vi "UI.vi"() -> ()   [LabVIEW 2018]
uses:
  data/MyControlAll.dll
panel:
  in  "多语言测试":refnum<k24>(container)
  in  "双击选中":refnum<k24>(container)
  in  "单击选中":refnum<k24>(container)
  in  "TreePanel":refnum<k24>(container)
  in  "按钮颜色":u32(colorbox)
  in  "渐变终点":u32(colorbox)
  in  "渐变起点":u32(colorbox)
  in  "ButtonPanel 10":refnum<k24>(container)
  in  "ButtonPanel 9":refnum<k24>(container)
  in  "开关":refnum<k24>(container)
  in  "文本":refnum<k24>(container)
  in  "滑动杆":refnum<k24>(container)
  in  "进度条":refnum<k24>(container)
  in  "ButtonPanel 4":refnum<k24>(container)
  in  "ButtonPanel 3":refnum<k24>(container)
  in  "ButtonPanel 2":refnum<k24>(container)
  in  "ButtonPanel":refnum<k24>(container)
  in  "ChartPanel":refnum<k24>(container)
  in  "DataGridPanel":refnum<k24>(container)
  in  "ButtonPanel 12":refnum<k24>(container)
  in  "ButtonPanel 11":refnum<k24>(container)
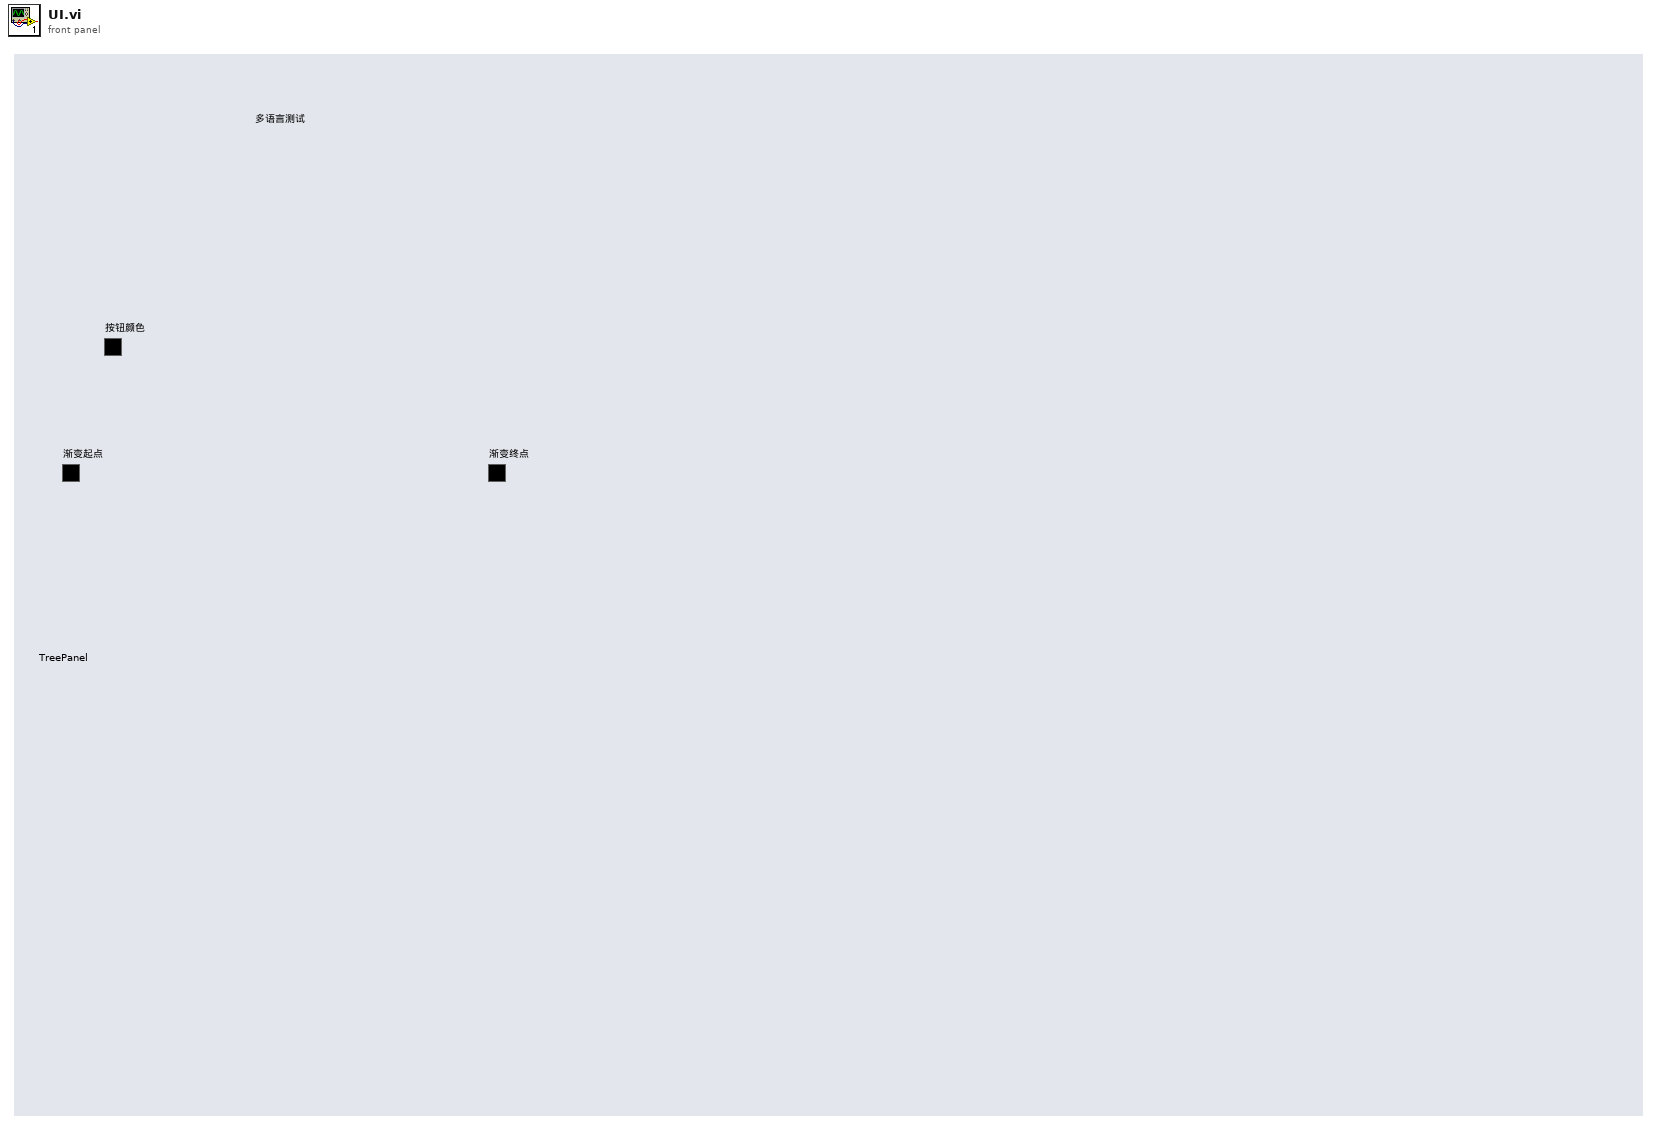
[diagram p1: front panel]
types:
  T1 = cluster{"selectedIndex":i32, "selectedItem":string, "selectedItemUTF8":u8[]}
  T2 = cluster{"nodeId":string, "nodeText":string, "nodeTextUTF8":u8[]}
  T3 = cluster{"id":string, "parentId":string, "text":string, "isChecked":bool, "showCheckBox":bool, "hasDummyChild":bool, "iconPath":string}[]
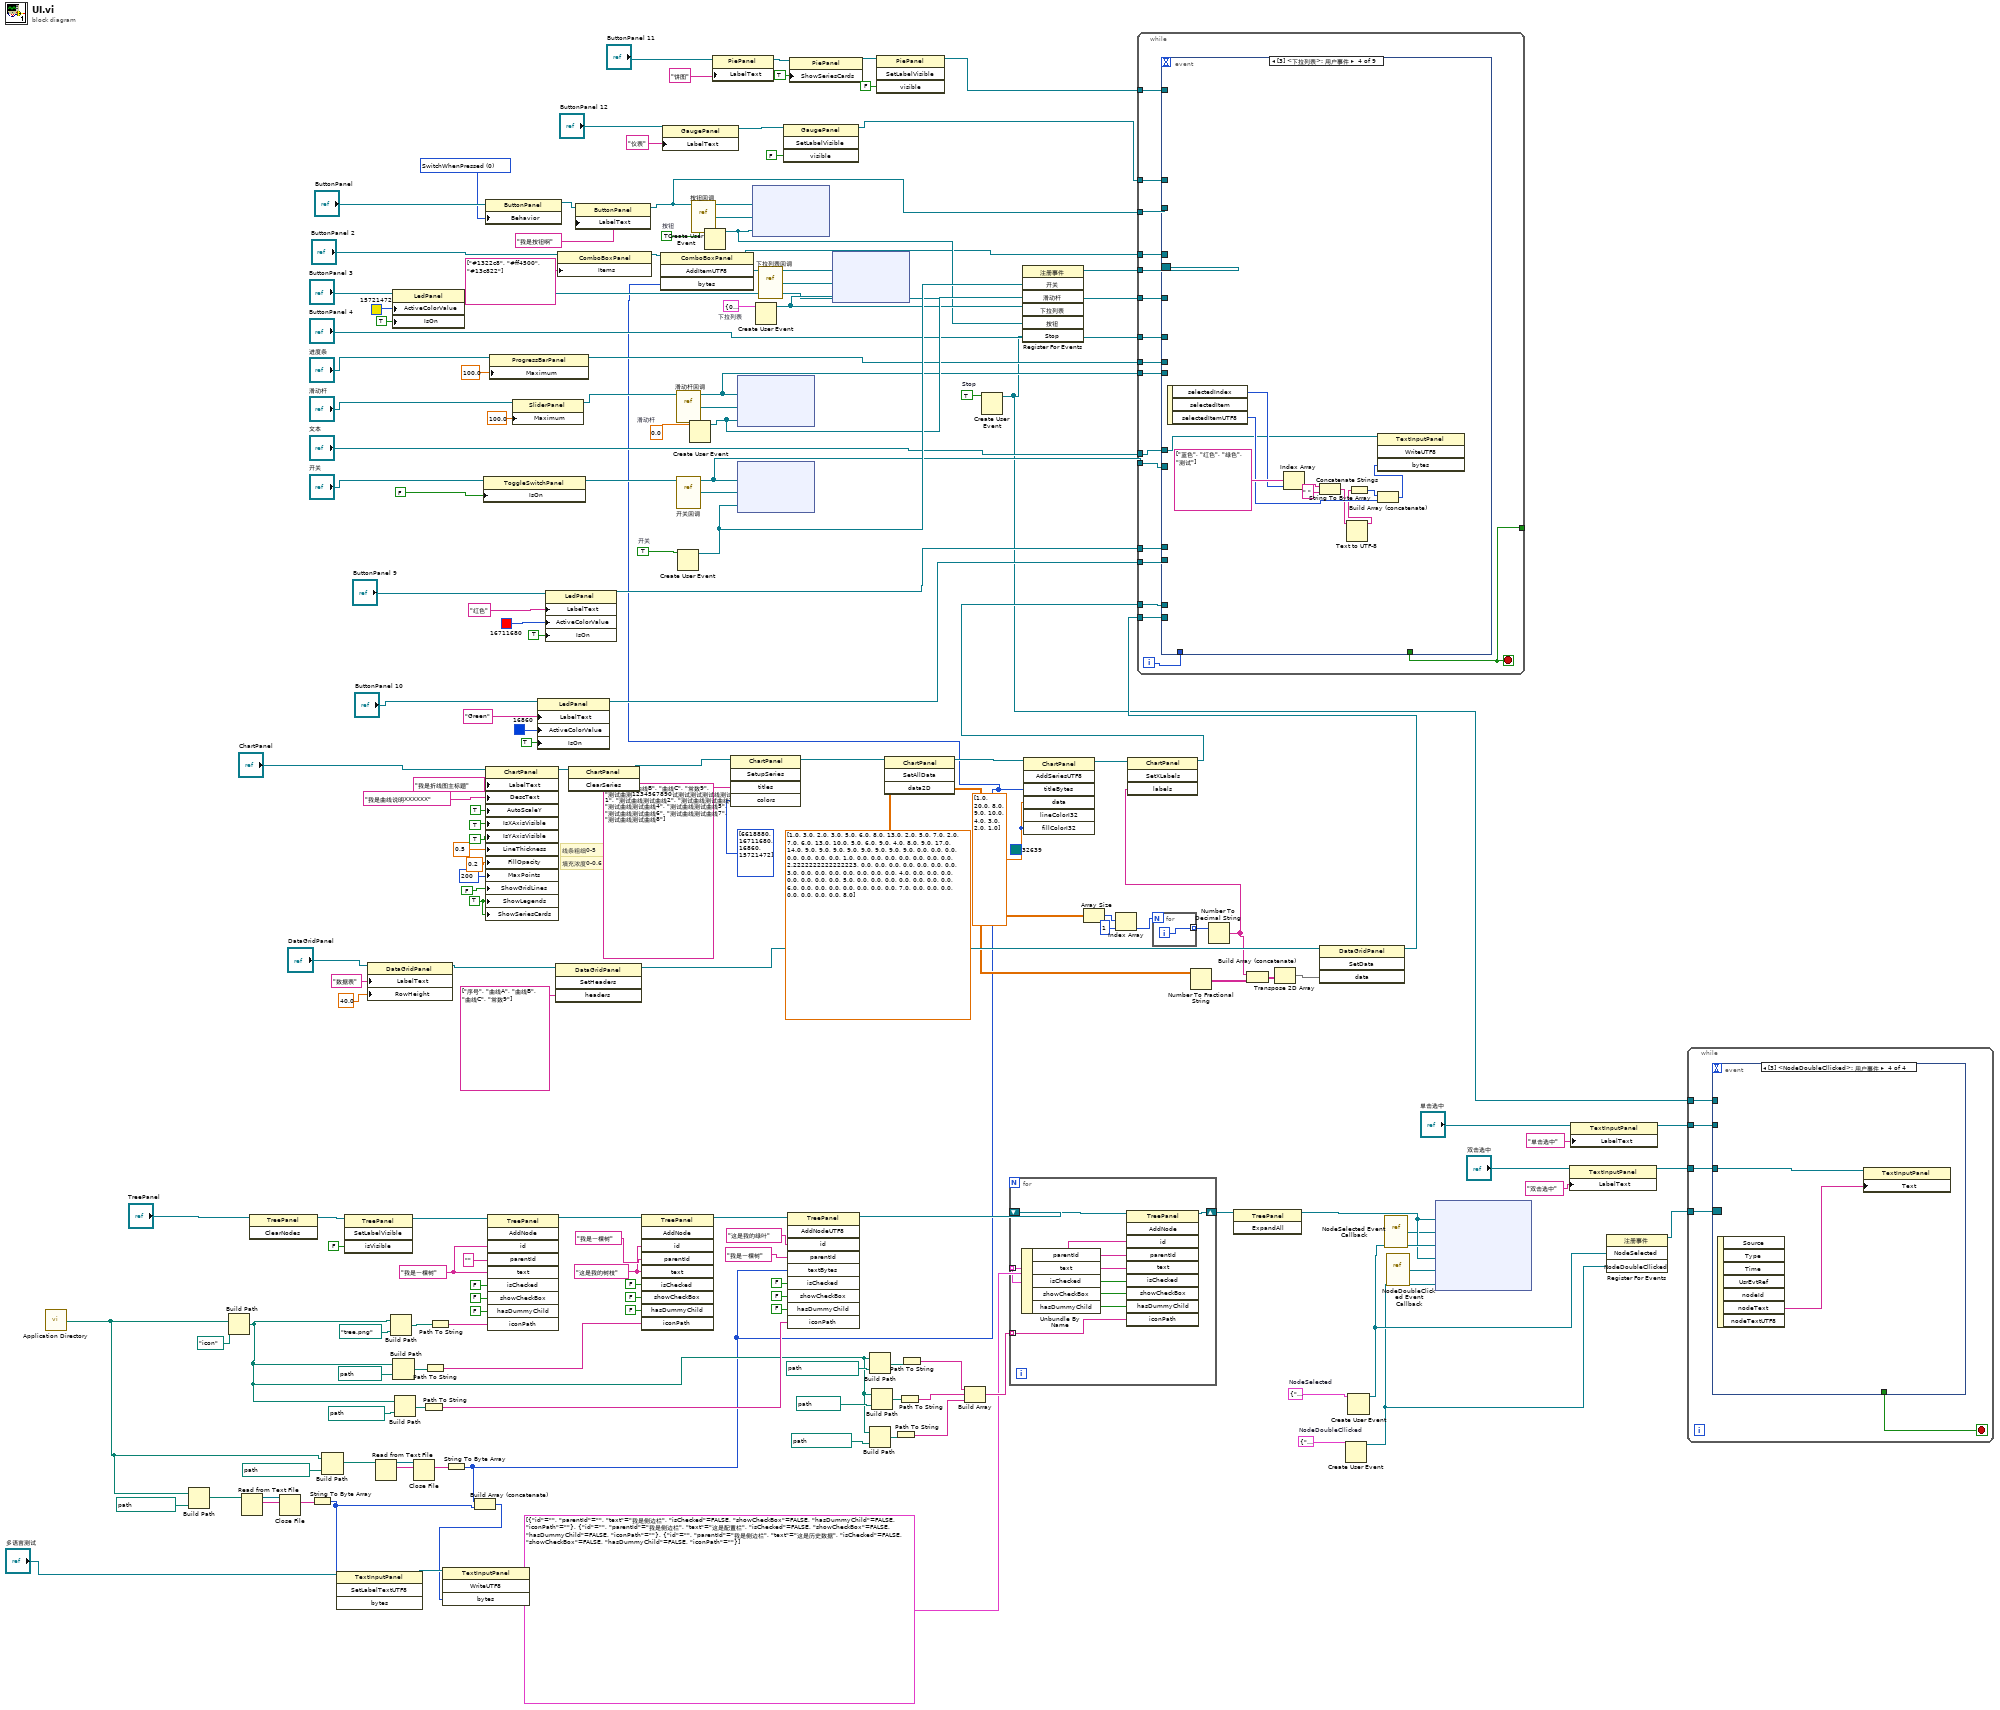
[diagram p0: block diagram]
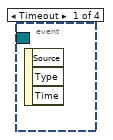
[diagram p2: hidden frame]
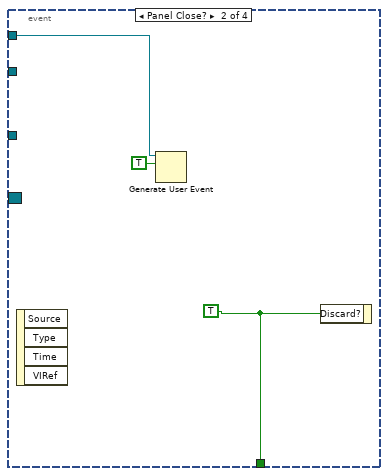
[diagram p3: hidden frame]
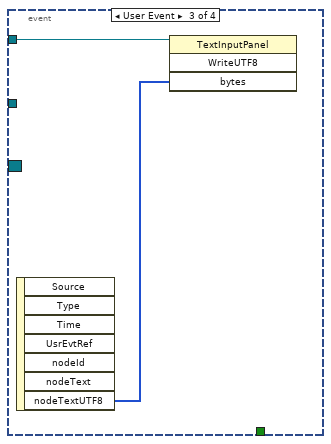
[diagram p4: hidden frame]
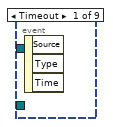
[diagram p5: hidden frame]
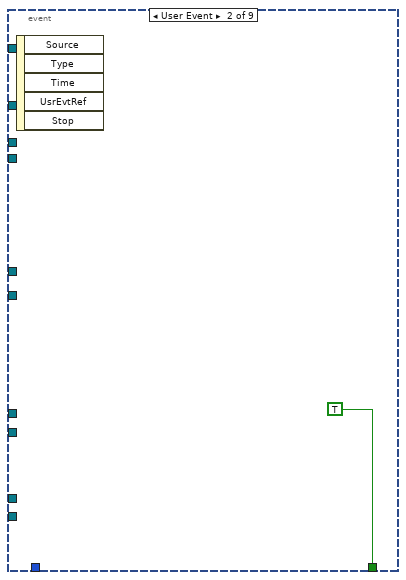
[diagram p6: hidden frame]
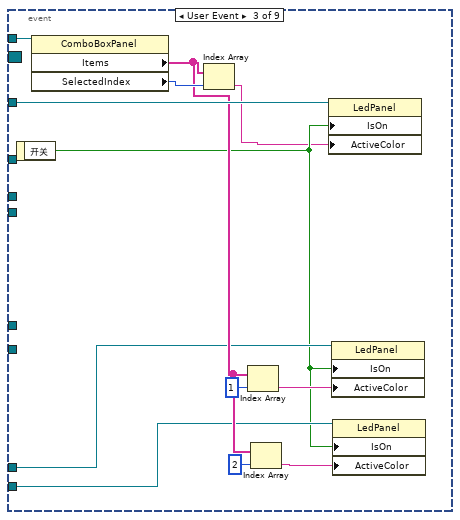
[diagram p7: hidden frame]
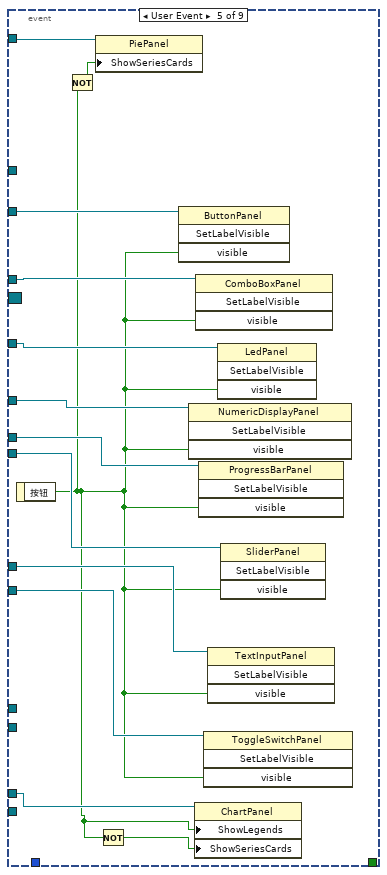
[diagram p8: hidden frame]
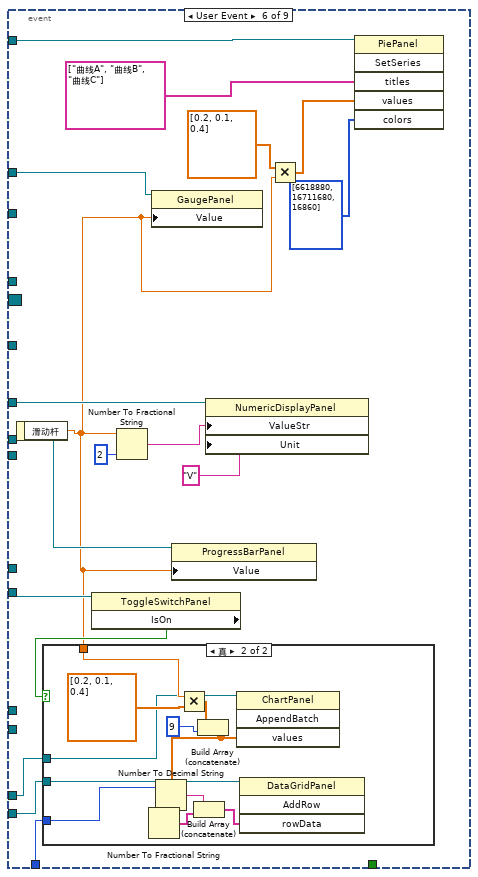
[diagram p9: hidden frame]
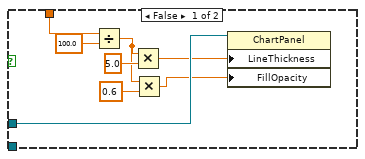
[diagram p10: hidden frame]
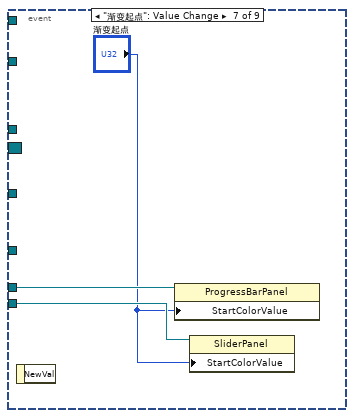
[diagram p11: hidden frame]
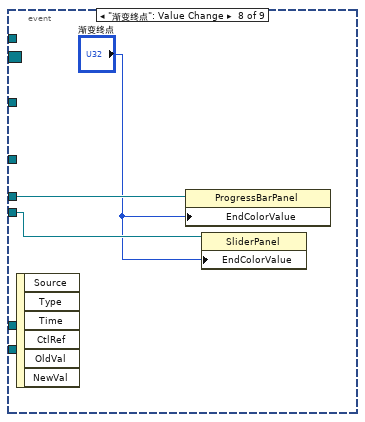
[diagram p12: hidden frame]
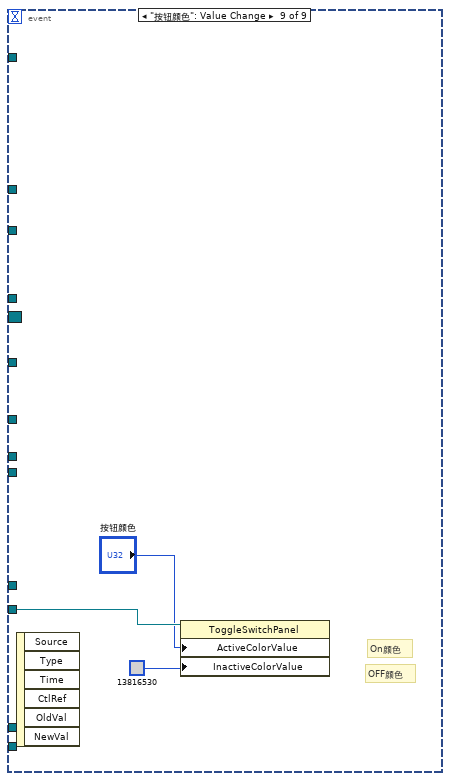
[diagram p13: hidden frame]
diagram:
  w3 = u32 32639
  w8 = T1 {"selectedIndex"=0, "selectedItem"="", "selectedItemUTF8"=[]}  # 下拉列表
  w11 = T2 {"nodeId"="", "nodeText"="", "nodeTextUTF8"=[]}  # NodeDoubleCllicked
  w12 = T2 {"nodeId"="", "nodeText"="", "nodeTextUTF8"=[]}  # NodeSelected
  w37 = TRUE  # Stop
  w63 = "这是我的树枝" ("text")
  w65 = "我是一棵树" ("text")
  w102 = TRUE ("ShowLegends")
  w141 = 0 items=["SwitchWhenPressed", "SwitchWhenReleased", "SwitchUntilReleased", "LatchWhenPressed", "LatchWhenReleased"] ("Behavior")
  w146 = TRUE  # 按钮
  w161 = 0.0  # 滑动杆
  w170 = TRUE  # 开关
  # "填充浓度0-0.6"
  # "线条粗细0-5"
  n1 = call <vilib>:"Application Directory.vi"() -> ("Application Directory"=w16:path)
  n2 = Build Path(base path=w16, name or relative path=path "data/韩文.txt" ("路径")) -> (appended path=w18:path)
  n3 = Build Path(base path=w16, name or relative path=path "icon" ("路径")) -> (appended path=w25:path)
  n4 = Read from Text File(file (use dialog)=w18) -> (refnum out=w20:refnum<file>, text=w19:string)  [unwired: 3 in, 2 out]
  n5 = invoke on="调用节点" class="TreePanel" method="ClearNodes"(reference="TreePanel") -> (reference out=w61:refnum<k24>)  [unwired: 2 in, 2 out]
  n6 = Close File(refnum=w20) -> ()  [unwired: 1 in, 2 out]
  n7 = String To Byte Array(string=w19) -> (unsigned byte array=w14:u8[])
  n8 = Build Path(base path=w16, name or relative path=path "data/越南文.txt" ("路径")) -> (appended path=w24:path)
  n9 = invoke on="调用节点" class="TextInputPanel" method="SetLabelTextUTF8"(reference="多语言测试", "bytes"=w14) -> (reference out=w15:refnum<k24>)  [unwired: 2 in, 3 out]
  n10 = invoke on="调用节点" class="TreePanel" method="SetLabelVisible"(reference=w61, "isVisible"=FALSE) -> (reference out=w59:refnum<k24>)  [unwired: 2 in, 3 out]
  n11 = property on="属性节点" class="DataGridPanel"(reference="DataGridPanel", "LabelText"="数据表", "RowHeight"=40.0) -> (reference out=w130:refnum<k24>)  [unwired: 1 in, 1 out]
  n12 = Read from Text File(file (use dialog)=w24) -> (refnum out=w22:refnum<file>, text=w23:string)  [unwired: 3 in, 2 out]
  n13 = Build Path(base path=w25, name or relative path=path "tree.png" ("路径")) -> (appended path=w48:path)
  n14 = property on="属性节点" class="LedPanel"(reference="ButtonPanel 3", "ActiveColorValue"=u32 15721472, "IsOn"=TRUE) -> (reference out=w97:refnum<k24>)  [unwired: 1 in, 1 out]
  n15 = Build Path(base path=w25, name or relative path=path "树枝.png" ("路径")) -> (appended path=w46:path)
  n16 = Build Path(base path=w25, name or relative path=path "绿叶 (1).png" ("路径")) -> (appended path=w44:path)
  n17 = Close File(refnum=w22) -> ()  [unwired: 1 in, 2 out]
  n18 = Path To String(path=w44) -> (string=w68:string)
  n19 = Path To String(path=w46) -> (string=w67:string)
  n20 = Path To String(path=w48) -> (string=w73:string)
  n21 = String To Byte Array(string=w23) -> (unsigned byte array=w1:u8[])
  n22 = Build Array (concatenate)(w1, w14) -> (w13:u8[])
  n23 = invoke on="调用节点" class="TextInputPanel" method="WriteUTF8"(reference=w15, "bytes"=w13) -> ()  [unwired: 2 in, 4 out]
  n24 = property on="属性节点" class="ToggleSwitchPanel"(reference="开关", "IsOn"=FALSE) -> (reference out=w140:refnum<k24>)  [unwired: 1 in, 1 out]
  n25 = property on="属性节点" class="ButtonPanel"(reference="ButtonPanel", "Behavior"=w141) -> (reference out=w138:refnum<k24>)  [unwired: 1 in, 1 out]
  n26 = property on="属性节点" class="ChartPanel"(reference="ChartPanel", "LabelText"="我是折线图主标题", "DescText"="我是曲线说明XXXXXX", "AutoScaleY"=TRUE, "IsXAxisVisible"=TRUE ("AutoScaleY"), "IsYAxisVisible"=TRUE ("AutoScaleY"), "LineThickness"=0.5, "FillOpacity"=0.2, "MaxPoints"=200, "ShowGridLines"=FALSE, "ShowLegends"=w102, "ShowSeriesCards"=w102) -> (reference out=w125:refnum<k24>)  [unwired: 1 in, 1 out]
  n27 = invoke on="调用节点" class="TreePanel" method="AddNode"(reference=w59, "id"=w65, "parentId"="", "text"=w65, "isChecked"=FALSE, "showCheckBox"=FALSE, "hasDummyChild"=FALSE, "iconPath"=w73) -> (reference out=w77:refnum<k24>)  [unwired: 2 in, 9 out]
  n28 = property on="属性节点" class="ProgressBarPanel"(reference="进度条", "Maximum"=100.0) -> (reference out=w155:refnum<k24>)  [unwired: 1 in, 1 out]
  n29 = property on="属性节点" class="SliderPanel"(reference="滑动杆", "Maximum"=100.0) -> (reference out=w139:refnum<k24>)  [unwired: 1 in, 1 out]
  n30 = property on="属性节点" class="LedPanel"(reference="ButtonPanel 10", "LabelText"="Green", "ActiveColorValue"=u32 16860, "IsOn"=TRUE) -> (reference out=w147:refnum<k24>)  [unwired: 1 in, 1 out]
  n31 = property on="属性节点" class="LedPanel"(reference="ButtonPanel 9", "LabelText"="红色", "ActiveColorValue"=u32 16711680, "IsOn"=TRUE) -> (reference out=w149:refnum<k24>)  [unwired: 1 in, 1 out]
  n32 = invoke on="调用节点" class="DataGridPanel" method="SetHeaders"(reference=w130, "headers"=string[] ["序号", "曲线A", "曲线B", "曲线C", "常数9"]) -> (reference out=w133:refnum<k24>)  [unwired: 2 in, 3 out]
  n33 = property class="ComboBoxPanel"(reference="ButtonPanel 2", "Items"=string[] ["#1322c8", "#ff4500", "#13c822"]) -> (reference out=w154:refnum<k24>)  [unwired: 1 in, 1 out]
  n34 = invoke on="调用节点" class="ChartPanel" method="ClearSeries"(reference=w125) -> (reference out=w111:refnum<k24>)  [unwired: 2 in, 2 out]
  n35 = property on="属性节点" class="ButtonPanel"(reference=w138, "LabelText"="我是按钮啊") -> (reference out=w137:refnum<k24>)  [unwired: 1 in, 1 out]
  n36 = invoke on="调用节点" class="TreePanel" method="AddNode"(reference=w77, "id"=w63, "parentId"="我是一棵树" ("text"), "text"=w63, "isChecked"=FALSE, "showCheckBox"=FALSE, "hasDummyChild"=FALSE, "iconPath"=w67) -> (reference out=w69:refnum<k24>)  [unwired: 2 in, 9 out]
  n37 = invoke on="调用节点" class="ComboBoxPanel" method="AddItemUTF8"(reference=w154, "bytes"=w1) -> (reference out=w2:refnum<k24>)  [unwired: 2 in, 3 out]
  n38 = property on="属性节点" class="GaugePanel"(reference="ButtonPanel 12", "LabelText"="仪表") -> (reference out=w90:refnum<k24>)  [unwired: 1 in, 1 out]
  n39 = vi-ref "滑动杆回调.vi"() -> ("vi reference"=w160:refnum<vi>)
  n40 = vi-ref "开关回调.vi"() -> ("vi reference"=w167:refnum<vi>)
  n41 = Create User Event(user event datatype=w170) -> (user event=w168:refnum<user-event>)  [unwired: 1 in, 1 out]
  n42 = Create User Event(user event datatype=w161) -> (user event=w159:refnum<user-event>)  [unwired: 1 in, 1 out]
  n43 = vi-ref "按钮回调.vi"() -> ("vi reference"=w144:refnum<vi>)
  n44 = Create User Event(user event datatype=w146) -> (user event=w143:refnum<user-event>)  [unwired: 1 in, 1 out]
  n45 = property on="属性节点" class="PiePanel"(reference="ButtonPanel 11", "LabelText"="饼图") -> (reference out=w85:refnum<k24>)  [unwired: 1 in, 1 out]
  n46 = invoke on="调用节点" class="ChartPanel" method="SetupSeries"(reference=w111, "titles"=string[] ["曲线A", "曲线B", "曲线C", "常数9", "测试曲测1234567890试测试测试测试线测试曲线1", "测试曲线测试曲线2", "测试曲线测试曲线3", "测试曲线测试曲线4", "测试曲线测试曲线5", "测试曲线测试曲线6", "测试曲线测试曲线7", "测试曲线测试曲线8"], "colors"=u32[] [6618880, 16711680, 16860, 15721472]) -> (reference out=w110:refnum<k24>)  [unwired: 2 in, 4 out]
  n47 = node(w139, w160, w159) -> ()  [unwired: 2 in, 2 out]
  n48 = node(w140, w167, w168) -> ()  [unwired: 2 in, 2 out]
  n49 = node(w137, w144, w143) -> ()  [unwired: 2 in, 2 out]
  n50 = Create User Event(user event datatype=w8) -> (user event=w153:refnum<user-event>)  [unwired: 1 in, 1 out]
  n51 = vi-ref "下拉列表回调.vi"() -> ("vi reference"=w7:refnum<vi>)
  n52 = invoke on="调用节点" class="GaugePanel" method="SetLabelVisible"(reference=w90, "visible"=FALSE) -> (reference out=w89:refnum<k24>)  [unwired: 2 in, 3 out]
  n53 = invoke on="调用节点" class="TreePanel" method="AddNodeUTF8"(reference=w69, "id"="这是我的绿叶" ("text"), "parentId"="我是一棵树" ("text"), "textBytes"=w1, "isChecked"=FALSE, "showCheckBox"=FALSE, "hasDummyChild"=FALSE, "iconPath"=w68) -> (reference out=w66:refnum<k24>)  [unwired: 2 in, 9 out]
  n54 = property on="属性节点" class="PiePanel"(reference=w85, "ShowSeriesCards"=TRUE) -> (reference out=w84:refnum<k24>)  [unwired: 1 in, 1 out]
  n55 = node(w2, w7, w153) -> ()  [unwired: 2 in, 2 out]
  n56 = Build Path(base path=w25, name or relative path=path "历史数据.png" ("路径")) -> (appended path=w38:path)
  n57 = Build Path(base path=w25, name or relative path=path "侧边栏_探索.png" ("路径")) -> (appended path=w42:path)
  n58 = Build Path(base path=w25, name or relative path=path "配置.png" ("路径")) -> (appended path=w40:path)
  n59 = invoke on="调用节点" class="PiePanel" method="SetLabelVisible"(reference=w84, "visible"=FALSE) -> (reference out=w87:refnum<k24>)  [unwired: 2 in, 3 out]
  n60 = invoke on="调用节点" class="ChartPanel" method="SetAllData"(reference=w110, "data2D"=dbl[][] [[1.0, 3.0, 2.0, 3.0, 5.0, 6.0, 8.0, 13.0], [2.0, 5.0, 7.0, 2.0, 7.0, 6.0, 13.0, 10.0], [5.0, 6.0, 9.0, 4.0, 8.0, 9.0, 17.0, 14.0], [9.0, 9.0, 9.0, 9.0, 9.0, 9.0, 9.0, 9.0], [0.0, 0.0, 0.0, 0.0, 0.0, 0.0, 0.0, 1.0], [0.0, 0.0, 0.0, 0.0, 0.0, 0.0, 0.0, 2.2222222222222223], [0.0, 0.0, 0.0, 0.0, 0.0, 0.0, 0.0, 3.0], [0.0, 0.0, 0.0, 0.0, 0.0, 0.0, 0.0, 4.0], [0.0, 0.0, 0.0, 0.0, 0.0, 0.0, 0.0, 5.0], [0.0, 0.0, 0.0, 0.0, 0.0, 0.0, 0.0, 6.0], [0.0, 0.0, 0.0, 0.0, 0.0, 0.0, 0.0, 7.0], [0.0, 0.0, 0.0, 0.0, 0.0, 0.0, 0.0, 8.0]]) -> (reference out=w6:refnum<k24>, "data2D"=w117:dbl[][])  [unwired: 2 in, 2 out]
  n61 = Path To String(path=w38) -> (string=w33:string)
  n62 = Path To String(path=w40) -> (string=w34:string)
  n63 = Path To String(path=w42) -> (string=w35:string)
  n64 = Build Array(w35, w34, w33) -> (w32:string[])
  n65 = Create User Event(user event datatype=w37) -> (user event=w36:refnum<user-event>)  [unwired: 1 in, 1 out]
  n66 = for {
    shift-right: [w180] -> w30
    shift-left: w66 -> [w181]
    tunnel: w32 -> [w179] mode=indexing
    tunnel: T3 [{"id"="", "parentId"="", "text"="我是侧边栏", "isChecked"=FALSE, "showCheckBox"=FALSE, "hasDummyChild"=FALSE, "iconPath"=""}, {"id"="", "parentId"="我是侧边栏", "text"="这是配置栏", "isChecked"=FALSE, "showCheckBox"=FALSE, "hasDummyChild"=FALSE, "iconPath"=""}, {"id"="", "parentId"="我是侧边栏", "text"="这是历史数据", "isChecked"=FALSE, "showCheckBox"=FALSE, "hasDummyChild"=FALSE, "iconPath"=""}] -> [w178] mode=indexing
    n67 = Unbundle By Name(w178) -> ("parentId"=w176:string, "text"=w177:string, "isChecked"=w175:bool, "showCheckBox"=w174:bool, "hasDummyChild"=w173:bool)
    n68 = invoke on="调用节点" class="TreePanel" method="AddNode"(reference=w181, "id"=w177, "parentId"=w176, "text"=w177, "isChecked"=w175, "showCheckBox"=w174, "hasDummyChild"=w173, "iconPath"=w179) -> (reference out=w180:refnum<k24>)  [unwired: 2 in, 9 out]
  }
  n69 = register-events(w168, w159, w153, w143, w36) -> (reference out=w169:refnum<event-registration>)  [unwired: 2 in, 1 out]
  n70 = invoke on="调用节点" class="ChartPanel" method="AddSeriesUTF8"(reference=w6, "titleBytes"=w1, "data"=dbl[] [1.0, 20.0, 8.0, 9.0, 10.0, 4.0, 3.0, 2.0, 1.0], "lineColorI32"=w3, "fillColorI32"=w3) -> (reference out=w5:refnum<k24>)  [unwired: 2 in, 6 out]
  n71 = Array Size(array=w117) -> (size(s)=w116:i32[])
  n72 = Index Array(array=w116, index=1 ("索引")) -> (element=w114:i32)
  n73 = for {
    N: w114 -> [_]
    tunnel: [w182] -> w113 mode=indexing
    i -> [w182]
  }
  n74 = Number To Fractional String(number=w117) -> (F-format string=w118:string[][])  [unwired: 3 in]
  n75 = Number To Decimal String(number=w113) -> (decimal integer string=w109:string[])  [unwired: 1 in]
  n76 = invoke on="调用节点" class="ChartPanel" method="SetXLabels"(reference=w5, "labels"=w109) -> (reference out=w108:refnum<k24>)  [unwired: 2 in, 3 out]
  n77 = invoke on="调用节点" class="TreePanel" method="ExpandAll"(reference=w30) -> (reference out=w29:refnum<k24>)  [unwired: 2 in, 2 out]
  n78 = Build Array (concatenate)(w109, w118) -> (w112:string[][])
  n79 = Transpose 2D Array(2D array=w112) -> (transposed array=w132:string[][])
  n80 = invoke on="调用节点" class="DataGridPanel" method="SetData"(reference=w133, "data"=w132) -> (reference out=w106:refnum<k24>)  [unwired: 2 in, 3 out]
  n81 = while {
    tunnel: w169 -> [w199]
    tunnel: w97 -> [w198]
    tunnel: w2 -> [w197]
    tunnel: "文本" -> [w196]
    tunnel: "ButtonPanel 4" -> [w195]
    tunnel: w155 -> [w194]
    tunnel: w149 -> [w193]
    tunnel: w147 -> [w192]
    tunnel: w137 -> [w191]
    tunnel: w140 -> [w190]
    tunnel: w139 -> [w189]
    tunnel: w108 -> [w188]
    tunnel: w106 -> [w187]
    tunnel: w89 -> [w185]
    tunnel: w87 -> [w184]
    tunnel: [w183] -> _
    i -> [w186]
    stop <- w183 stop-if-true
    n82 = event shown="[3] <下拉列表>: 用户事件" {
      selector: w199 -> [_ _ _ _ _ _ _ _ _]
      dyn-events: _ -> [_ _ _ _ _ _ _ _ _]
      timeout: _ -> [_ _ _ _ _ _ _ _ _]
      tunnel: [_ TRUE _ _ _ _ _ _ _] -> w183
      tunnel: w198 -> [_ _ w212 _ w234 _ _ _ _]
      tunnel: w197 -> [_ _ w211 _ w235 _ _ _ _]
      tunnel: w196 -> [_ _ _ w216 w231 _ _ _ _]
      tunnel: w195 -> [_ _ _ _ w233 w252 _ _ _]
      tunnel: w194 -> [_ _ _ _ w232 w248 w274 w277 _]
      tunnel: w193 -> [_ _ w208 _ _ _ _ _ _]
      tunnel: w192 -> [_ _ w206 _ _ _ _ _ _]
      tunnel: w191 -> [_ _ _ _ w230 _ _ _ _]
      tunnel: w190 -> [_ _ _ _ w229 w246 _ _ w280]
      tunnel: w189 -> [_ _ _ _ w228 _ w273 w276 _]
      tunnel: w188 -> [_ _ _ _ w227 w247 _ _ _]
      tunnel: w187 -> [_ _ _ _ _ w244 _ _ _]
      tunnel: w186 -> [_ _ _ _ _ w243 _ _ _]
      tunnel: w185 -> [_ _ _ _ _ w242 _ _ _]
      tunnel: w184 -> [_ _ _ _ w225 w241 _ _ _]
      event Timeout {
        n83 = event-data() -> ()  [unwired: 1 in, 3 out]
      }
      event User Event {
        n84 = event-data() -> ()  [unwired: 1 in, 5 out]
      }
      event User Event {
        n85 = event-data() -> ("开关"=w205:bool)  [unwired: 1 in]
        n86 = property class="ComboBoxPanel"(reference=w211) -> ("Items"=w209:string[], "SelectedIndex"=w210:i32)  [unwired: 1 in, 2 out]
        n87 = Index Array(array=w209, index=w210) -> (element=w201:string)
        n88 = Index Array(array=w209, index=1 ("索引")) -> (element=w207:string)
        n89 = Index Array(array=w209, index=2 ("索引")) -> (element=w204:string)
        n90 = property on="属性节点" class="LedPanel"(reference=w212, "IsOn"=w205, "ActiveColor"=w201) -> ()  [unwired: 1 in, 2 out]
        n91 = property on="属性节点" class="LedPanel"(reference=w208, "IsOn"=w205, "ActiveColor"=w207) -> ()  [unwired: 1 in, 2 out]
        n92 = property on="属性节点" class="LedPanel"(reference=w206, "IsOn"=w205, "ActiveColor"=w204) -> ()  [unwired: 1 in, 2 out]
      }
      event User Event {
        n93 = event-data() -> ("selectedIndex"=w221:i32, "selectedItemUTF8"=w217:u8[])  [unwired: 1 in, 1 out]
        n94 = Index Array(array=string[] ["蓝色", "红色", "绿色", "测试"], index=w221) -> (element=w220:string)
        n95 = Concatenate Strings(w220, " " ("字符串")) -> (w214:string)
        n96 = Text to UTF-8(11:w214) -> (3:w213:string)  [unwired: 2 in, 1 out]
        n97 = String To Byte Array(string=w213) -> (unsigned byte array=w218:u8[])
        n98 = Build Array (concatenate)(w218, w217) -> (w215:u8[])
        n99 = invoke on="调用节点" class="TextInputPanel" method="WriteUTF8"(reference=w216, "bytes"=w215) -> ()  [unwired: 2 in, 4 out]
      }
      event User Event {
        n100 = event-data() -> ("按钮"=w224:bool)  [unwired: 1 in]
        n101 = Not(x=w224) -> (.not. x?=w223:bool)
        n102 = property on="属性节点" class="PiePanel"(reference=w225, "ShowSeriesCards"=w223) -> ()  [unwired: 1 in, 2 out]
        n103 = Not(x=w224) -> (.not. x?=w226:bool)
        n104 = invoke on="调用节点" class="ButtonPanel" method="SetLabelVisible"(reference=w230, "visible"=w224) -> ()  [unwired: 2 in, 4 out]
        n105 = invoke on="调用节点" class="NumericDisplayPanel" method="SetLabelVisible"(reference=w233, "visible"=w224) -> ()  [unwired: 2 in, 4 out]
        n106 = property on="属性节点" class="ChartPanel"(reference=w227, "ShowLegends"=w224, "ShowSeriesCards"=w226) -> ()  [unwired: 1 in, 2 out]
        n107 = invoke on="调用节点" class="ComboBoxPanel" method="SetLabelVisible"(reference=w235, "visible"=w224) -> ()  [unwired: 2 in, 4 out]
        n108 = invoke on="调用节点" class="ProgressBarPanel" method="SetLabelVisible"(reference=w232, "visible"=w224) -> ()  [unwired: 2 in, 4 out]
        n109 = invoke on="调用节点" class="ToggleSwitchPanel" method="SetLabelVisible"(reference=w229, "visible"=w224) -> ()  [unwired: 2 in, 4 out]
        n110 = invoke on="调用节点" class="TextInputPanel" method="SetLabelVisible"(reference=w231, "visible"=w224) -> ()  [unwired: 2 in, 4 out]
        n111 = invoke on="调用节点" class="LedPanel" method="SetLabelVisible"(reference=w234, "visible"=w224) -> ()  [unwired: 2 in, 4 out]
        n112 = invoke on="调用节点" class="SliderPanel" method="SetLabelVisible"(reference=w228, "visible"=w224) -> ()  [unwired: 2 in, 4 out]
      }
      event User Event {
        n113 = event-data() -> ("滑动杆"=w238:dbl)  [unwired: 1 in]
        n114 = property on="属性节点" class="ToggleSwitchPanel"(reference=w246) -> ("IsOn"=w245:bool)  [unwired: 1 in, 2 out]
        n115 = case shown="真" w245 {
          tunnel: w247 -> [w260 w269]
          tunnel: w238 -> [w259 w270]
          tunnel: w244 -> [_ w268]
          tunnel: w243 -> [_ w265]
          frame False {
            n116 = Divide(x=w259, y=100.0) -> (x/y=w255:dbl)
            n117 = Multiply(x=w255, y=5.0) -> (x*y=w256:dbl)
            n118 = Multiply(x=w255, y=0.6) -> (x*y=w253:dbl)
            n119 = property on="属性节点" class="ChartPanel"(reference=w260, "LineThickness"=w256, "FillOpacity"=w253) -> ()  [unwired: 1 in, 2 out]
          }
          frame True {
            n120 = Number To Decimal String(number=w265) -> (decimal integer string=w264:string)  [unwired: 1 in]
            n121 = Multiply(x=w270, y=dbl[] [0.2, 0.1, 0.4]) -> (x*y=w267:dbl[])
            n122 = Build Array (concatenate)(w267, 9) -> (w262:dbl[])
            n123 = Number To Fractional String(number=w262) -> (F-format string=w266:string[])  [unwired: 3 in]
            n124 = Build Array (concatenate)(w264, w266) -> (w263:string[])
            n125 = invoke on="调用节点" class="ChartPanel" method="AppendBatch"(reference=w269, "values"=w262) -> ()  [unwired: 2 in, 4 out]
            n126 = invoke on="调用节点" class="DataGridPanel" method="AddRow"(reference=w268, "rowData"=w263) -> ()  [unwired: 2 in, 4 out]
          }
        }
        n127 = Number To Fractional String(number=w238, precision (6)=i16 2 ("精度(6)")) -> (F-format string=w250:string)  [unwired: 2 in]
        n128 = property on="属性节点" class="GaugePanel"(reference=w242, "Value"=w238) -> ()  [unwired: 1 in, 2 out]
        n129 = property on="属性节点" class="ProgressBarPanel"(reference=w248, "Value"=w238) -> ()  [unwired: 1 in, 2 out]
        n130 = property on="属性节点" class="NumericDisplayPanel"(reference=w252, "ValueStr"=w250, "Unit"="V") -> ()  [unwired: 1 in, 2 out]
        n131 = Multiply(x=dbl[] [0.2, 0.1, 0.4], y=w238) -> (x*y=w237:dbl[])
        n132 = invoke on="调用节点" class="PiePanel" method="SetSeries"(reference=w241, "titles"=string[] ["曲线A", "曲线B", "曲线C"], "values"=w237, "colors"=u32[] [6618880, 16711680, 16860]) -> ()  [unwired: 2 in, 6 out]
      }
      event "渐变起点": Value Change {
        n133 = event-data() -> ()  [unwired: 1 in, 1 out]
        n134 = property on="属性节点" class="ProgressBarPanel"(reference=w274, "StartColorValue"="渐变起点") -> ()  [unwired: 1 in, 2 out]
        n135 = property on="属性节点" class="SliderPanel"(reference=w273, "StartColorValue"="渐变起点") -> ()  [unwired: 1 in, 2 out]
      }
      event "渐变终点": Value Change {
        n136 = event-data() -> ()  [unwired: 1 in, 6 out]
        n137 = property on="属性节点" class="ProgressBarPanel"(reference=w277, "EndColorValue"="渐变终点") -> ()  [unwired: 1 in, 2 out]
        n138 = property on="属性节点" class="SliderPanel"(reference=w276, "EndColorValue"="渐变终点") -> ()  [unwired: 1 in, 2 out]
      }
      event "按钮颜色": Value Change {
        # "OFF颜色"
        # "On颜色"
        n139 = event-data() -> ()  [unwired: 1 in, 6 out]
        n140 = property on="属性节点" class="ToggleSwitchPanel"(reference=w280, "ActiveColorValue"="按钮颜色", "InactiveColorValue"=u32 13816530) -> ()  [unwired: 1 in, 2 out]
      }
    }
  }
  n141 = Create User Event(user event datatype=w11) -> (user event=w57:refnum<user-event>)  [unwired: 1 in, 1 out]
  n142 = Create User Event(user event datatype=w12) -> (user event=w58:refnum<user-event>)  [unwired: 1 in, 1 out]
  n143 = vi-ref "NodeSelected Event Callback.vi"() -> ("vi reference"=w10:refnum<vi>)
  n144 = vi-ref "NodeDoubleClicked Event Callback.vi"() -> ("vi reference"=w9:refnum<vi>)
  n145 = node(w29, w10, w58, w29, w9, w57) -> ()  [unwired: 2 in, 2 out]
  n146 = property on="属性节点" class="TextInputPanel"(reference="双击选中", "LabelText"="双击选中") -> (reference out=w50:refnum<k24>)  [unwired: 1 in, 1 out]
  n147 = property on="属性节点" class="TextInputPanel"(reference="单击选中", "LabelText"="单击选中") -> (reference out=w51:refnum<k24>)  [unwired: 1 in, 1 out]
  n148 = register-events(w58, w57) -> (reference out=w56:refnum<event-registration>)  [unwired: 2 in, 1 out]
  n149 = while {
    tunnel: w56 -> [w284]
    tunnel: w51 -> [w283]
    tunnel: w50 -> [w282]
    tunnel: w36 -> [w281]
    stop <- w285 stop-if-true
    n150 = event shown="[3] <NodeDoubleCllicked>: 用户事件" {
      selector: w284 -> [_ _ _ _]
      dyn-events: _ -> [_ _ _ _]
      timeout: _ -> [_ _ _ _]
      tunnel: [_ w288 _ _] -> w285
      tunnel: w283 -> [_ _ w290 _]
      tunnel: w282 -> [_ _ _ w292]
      tunnel: w281 -> [_ w287 _ _]
      event Timeout {
        n151 = event-data() -> ()  [unwired: 1 in, 3 out]
      }
      event Panel Close? {
        w288 = TRUE
        n152 = event-data() -> ()  [unwired: 1 in, 4 out]
        n153 = Generate User Event(user event=w287, event data cluster=TRUE ("事件数据")) -> ()  [unwired: 2 in, 2 out]
        n154 = event-data("Discard?"=w288) -> ()  [unwired: 1 in, 1 out]
      }
      event User Event {
        n155 = event-data() -> ("nodeTextUTF8"=w289:u8[])  [unwired: 1 in, 6 out]
        n156 = invoke on="调用节点" class="TextInputPanel" method="WriteUTF8"(reference=w290, "bytes"=w289) -> ()  [unwired: 2 in, 4 out]
      }
      event User Event {
        n157 = event-data() -> ("nodeText"=w291:string)  [unwired: 1 in, 6 out]
        n158 = property class="TextInputPanel"(reference=w292, "Text"=w291) -> ()  [unwired: 1 in, 2 out]
      }
    }
  }
